vi "Log Double Data.vi"(0 "TDMS Data Logger Actor in":refnum<class "TDMS Data Logger Actor.lvclass">, 5 "Group Name":string, 7 "Channel Names (Untitled)":string[](array[string]), 9 "Data":dbl[][](array[numeric]), 11 "error in (no error)":errorcluster) -> (4 "TDMS Data Logger Actor out":refnum<class "TDMS Data Logger Actor.lvclass">, 15 "error out":errorcluster)   [LabVIEW 2024, in "TDMS Data Logger Actor.lvlib" / "TDMS Data Logger Actor.lvclass"]
uses:
  TDMS Data Logger Actor.lvclass
  TDMS Data Logger Actor.lvclass/TDMS Data Logger Actor.ctl
  Logging Data/2D Double Data/2D Double Logging Data.lvclass
  C:/Users/uspoaotto/OneDrive - Oregon Tool/Desktop/working copies/dataLogger/Logging Data Interface/Logging Data Interface/Logging Data Interface.lvclass
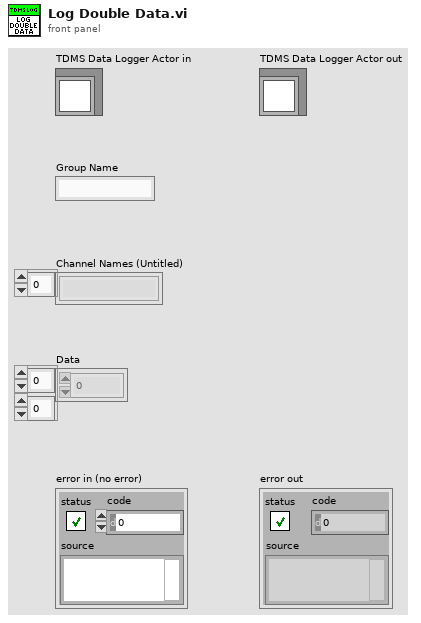
[diagram p1: front panel]
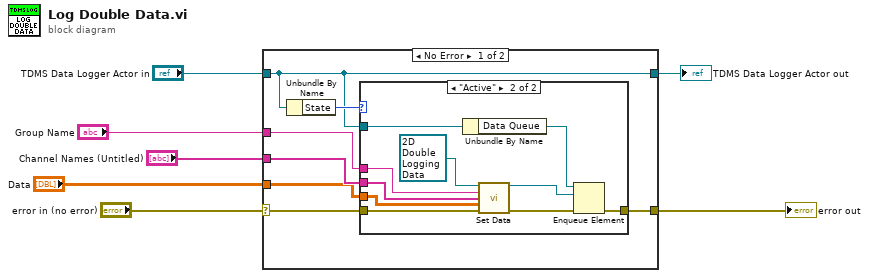
[diagram p0: block diagram]
diagram:
  n1 = case shown="No Error" "error in (no error)" {
    selector: "error in (no error)" -> [w11 w26]
    tunnel: "TDMS Data Logger Actor in" -> [w13 w27]
    tunnel: "Channel Names (Untitled)" -> [w9 _]
    tunnel: "Group Name" -> [w10 _]
    tunnel: "Data" -> [w8 _]
    tunnel: [w13 w27] -> w3
    tunnel: [w12 w26] -> w2
    frame No Error {
      n2 = Unbundle By Name(w13) -> ("State"=w14:enum16{"Idle", "Active", "Paused"})
      n3 = case shown="\"Active\"" w14 {
        tunnel: w13 -> [_ w25]
        tunnel: [w15 w23] -> w12
        tunnel: w11 -> [w15 w19]
        tunnel: w10 -> [_ w22]
        tunnel: w9 -> [_ w21]
        tunnel: w8 -> [_ w20]
        frame "Idle", "Paused" {
        }
        frame "Active" {
          n4 = Unbundle By Name(w25) -> ("Data Queue"=w24:refnum<queue>)
          n5 = call-dynamic "Set Data.vi"("2D Double Data in"=refnum<class "2D Double Logging Data.lvclass"> refnum, "Group Name"=w22, "Channel Names"=w21, "Data"=w20, "error in (no error)"=w19) -> ("2D Double Data out"=w16:refnum<class "2D Double Logging Data.lvclass">, "error out"=w18:errorcluster)  [unwired: 9 in]
          n6 = Enqueue Element(queue=w24, element=w16, error in (no error)=w18) -> (error out=w23:errorcluster)  [unwired: 1 in, 2 out]
        }
      }
    }
    frame Error {
    }
  }
  "error out" <- w2
  "TDMS Data Logger Actor out" <- w3
